vi "Populate Plugin Tree.vi"(8 "ErrorArray In":errorcluster[](array[cluster]), 10 "Userfiles Directory":path, 11 "PluginTreeRef":refnum<vi>) -> (0 "ErrorArray Out":errorcluster[](array[cluster]), 2 "All Tags":string[](array[string]), 3 "Tree Ref out":refnum<vi>)   [LabVIEW 2018]
uses:
  Controls/Plugins Tree Item Type.ctl
  <userlib>/NIST/NISTErrorLib/NISTErrorLib.lvlib
panel:
  in  "PluginTree":string(tree)
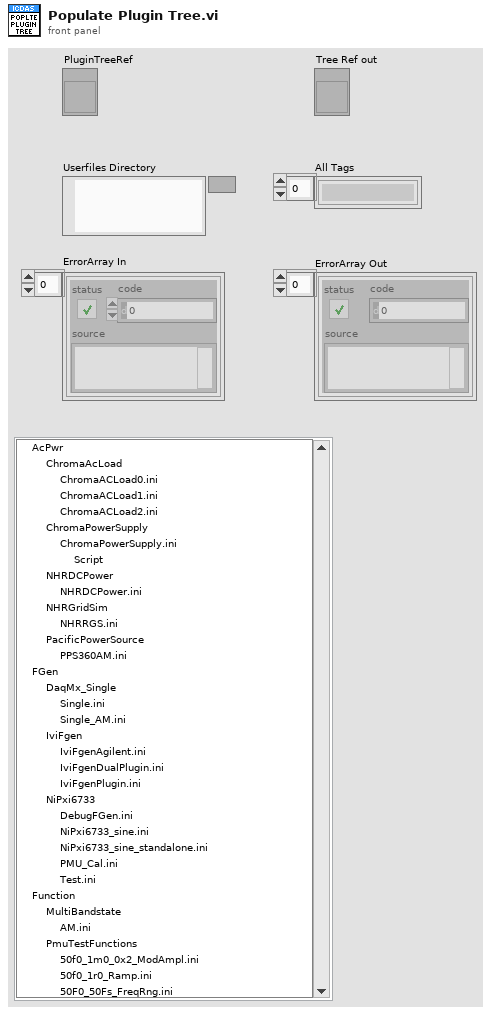
[diagram p1: front panel]
types:
  T1 = typedef "Plugins Tree Item Type.ctl" = enum16{"Plugin", "Instrument", "INI File", "INI Script"}
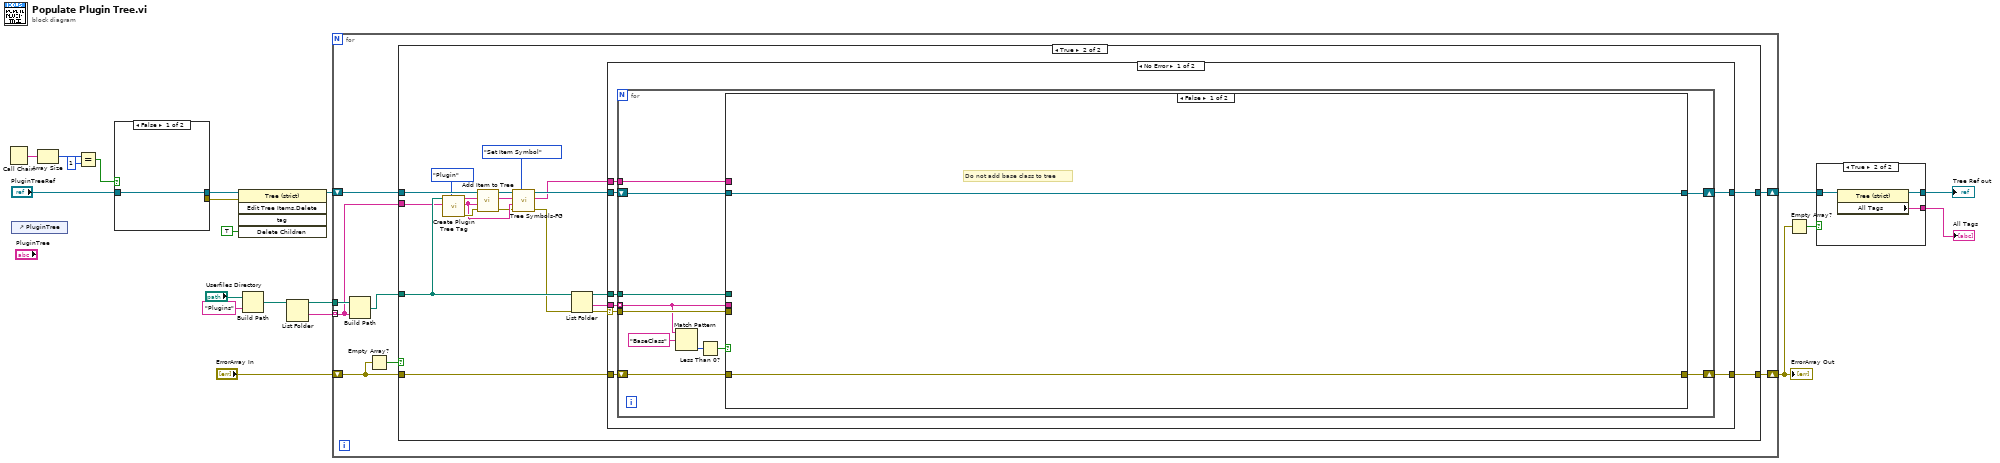
[diagram p0: block diagram]
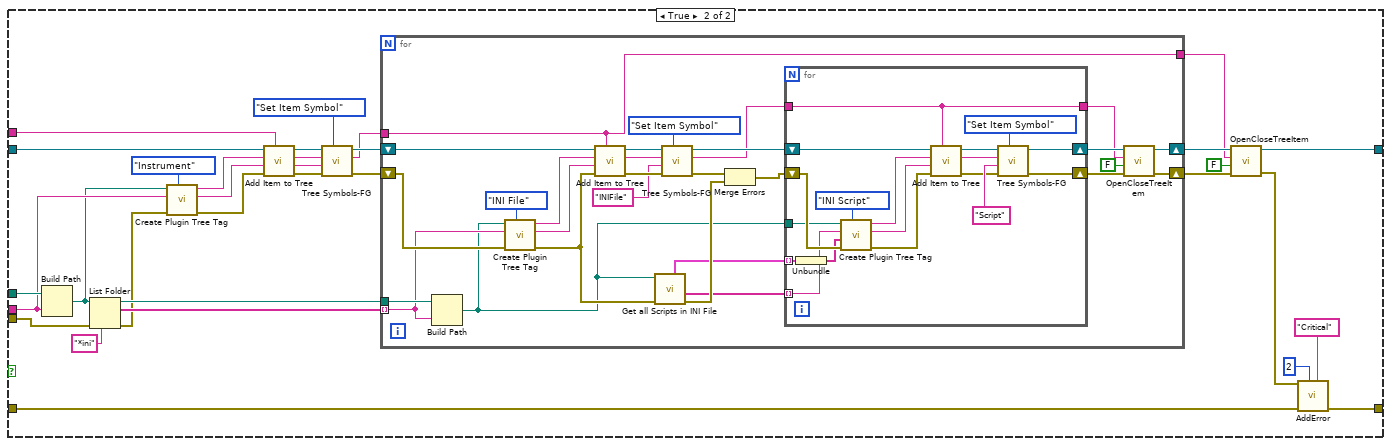
[diagram p4: hidden frame]
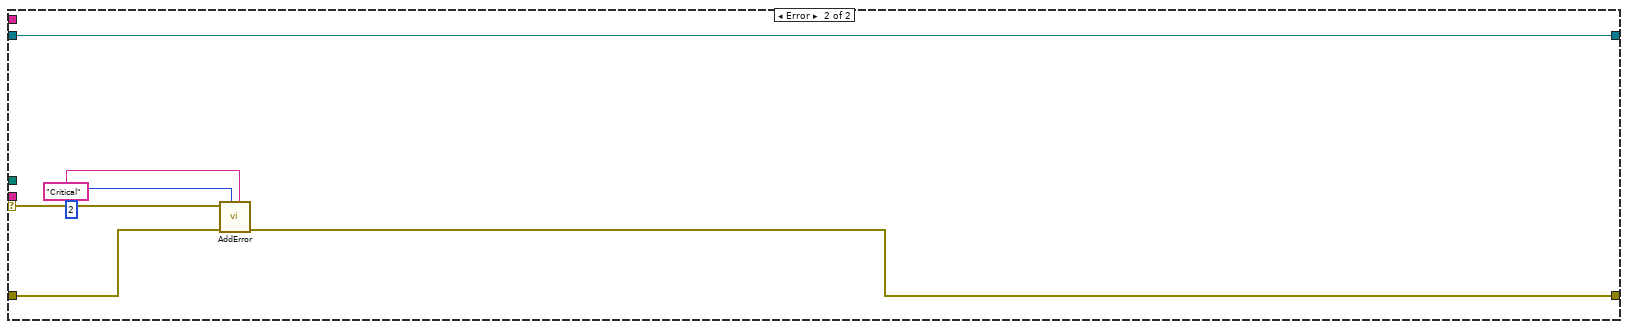
[diagram p5: hidden frame]
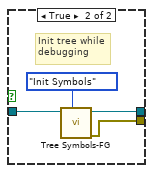
[diagram p6: hidden frame]
diagram:
  n1 = Call Chain() -> (call chain=w13:string[])
  n2 = control-ref of="PluginTree"() -> ()  [unwired: 1 out]
  n3 = Array Size(array=w13) -> (size(s)=w12:i32)
  n4 = Equal?(x=w12, y=1) -> (x = y?=w10:bool)
  n5 = case shown="False" w10 {
    tunnel: [w21 w24] -> w15
    tunnel: "PluginTreeRef" -> [w21 w23]
    tunnel: [_ w22] -> w14
    frame False {
    }
    frame True {
      # "Init tree while\ndebugging"
      n6 = call "Tree Symbols-FG.vi"("Actions"=enum16{"Init Symbols", "Set Item Symbol"}."Init Symbols", "Tree Ref"=w23) -> ("error out"=w22:errorcluster, "Tree Ref out"=w24:refnum<vi>)  [unwired: 7 in, 1 out]
    }
  }
  n7 = invoke class="Tree (strict)" method="Edit Tree Items.Delete"(reference=w15, error in=w14, "Delete Children"=TRUE ("Delete Children?")) -> (reference out=w17:refnum<vi>)  [unwired: 2 in, 4 out]
  n8 = Build Path(base path="Userfiles Directory", name or relative path="Plugins") -> (appended path=w1:path)
  n9 = List Folder(path=w1) -> (path out=w19:path, folder names=w20:string[])  [unwired: 3 in, 2 out]
  n10 = for {
    tunnel: w20 -> [w26] mode=indexing
    tunnel: w19 -> [w33]
    shift-right: [w30] -> w6
    shift-left: "ErrorArray In" -> [w31]
    shift-right: [w28] -> w8
    shift-left: w17 -> [w29]
    n11 = Build Path(base path=w33, name or relative path=w26) -> (appended path=w32:path)
    n12 = Empty Array?(array=w31) -> (empty?=w27:bool)
    n13 = case shown="True" w27 {
      tunnel: w32 -> [_ w47]
      tunnel: w31 -> [w34 w55]
      tunnel: [w34 w54] -> w30
      tunnel: w29 -> [w35 w49]
      tunnel: [w35 w50] -> w28
      tunnel: w26 -> [_ w46]
      frame False {
      }
      frame True {
        n14 = call "Create Plugin Tree Tag.vi"("ItemType"=Plugins_Tree_Item_Type."Plugin", "Name"=w46, "VISA Resource"=w47) -> ("error out"=w44:errorcluster, "Name out"=w38:string, "Tag"=w45:string)  [unwired: 6 in]
        n15 = call "Add Item to Tree.vi"("error in (no error)"=w44, "Item Name"=w38, "Item Tag"=w45, "Tree Ref"=w49) -> ("error out"=w37:errorcluster, "Item Tag out"=w40:string, "reference out"=w48:refnum<vi>)  [unwired: 4 in, 1 out]
        n16 = call "Tree Symbols-FG.vi"("Actions"=enum16{"Init Symbols", "Set Item Symbol"}."Set Item Symbol", "error in (no error)"=w37, "Symbol Name"=w38, "Item Tag"=w40, "Tree Ref"=w48) -> ("error out"=w36:errorcluster, "Item Tag out"=w39:string, "Tree Ref out"=w42:refnum<vi>)  [unwired: 4 in]
        n17 = List Folder(path=w47, error in=w36) -> (path out=w51:path, folder names=w52:string[], error out=w53:errorcluster)  [unwired: 2 in, 1 out]
        n18 = case shown="No Error" w53 {
          selector: w53 -> [w56 w159]
          tunnel: w55 -> [w61 w160]
          tunnel: [w60 w156] -> w54
          tunnel: w52 -> [w63 _]
          tunnel: w51 -> [w62 _]
          tunnel: w42 -> [w59 w155]
          tunnel: [w58 w155] -> w50
          tunnel: w39 -> [w57 _]
          frame No Error {
            n19 = for {
              tunnel: w63 -> [w67] mode=indexing
              tunnel: w62 -> [w74]
              shift-right: [w72] -> w60
              shift-left: w61 -> [w73]
              shift-right: [w68] -> w58
              shift-left: w59 -> [w71]
              tunnel: w57 -> [w70]
              tunnel: w56 -> [w69]
              n20 = Match Pattern(string=w67, regular expression="BaseClass") -> (offset past match=w65:i32)  [unwired: 1 in, 3 out]
              n21 = Less Than 0?(x=w65) -> (x < 0?=w64:bool)
              n22 = case shown="False" w64 {
                tunnel: w74 -> [_ w106]
                tunnel: w73 -> [w76 w104]
                tunnel: [w76 w103] -> w72
                tunnel: w71 -> [w75 w100]
                tunnel: w70 -> [_ w99]
                tunnel: w67 -> [_ w98]
                tunnel: w69 -> [_ w91]
                tunnel: [w75 w81] -> w68
                frame False {
                  # "Do not add base class to tree"
                }
                frame True {
                  n23 = Build Path(base path=w106, name or relative path=w98) -> (appended path=w97:path)
                  n24 = List Folder(path=w97, pattern="*ini", error in=w91) -> (path out=w105:path, filenames=w107:string[], error out=w90:errorcluster)  [unwired: 1 in, 1 out]
                  n25 = call "Create Plugin Tree Tag.vi"("ItemType"=Plugins_Tree_Item_Type."Instrument", "error in (no error)"=w90, "Name"=w98, "VISA Resource"=w97) -> ("error out"=w93:errorcluster, "Name out"=w94:string, "Tag"=w95:string)  [unwired: 5 in]
                  n26 = call "Add Item to Tree.vi"("Parent Tag"=w99, "error in (no error)"=w93, "Item Name"=w94, "Item Tag"=w95, "Tree Ref"=w100) -> ("error out"=w92:errorcluster, "Item Name out"=w83:string, "Item Tag out"=w86:string, "reference out"=w88:refnum<vi>)  [unwired: 3 in]
                  n27 = call "Tree Symbols-FG.vi"("Actions"=enum16{"Init Symbols", "Set Item Symbol"}."Set Item Symbol", "error in (no error)"=w92, "Symbol Name"=w83, "Item Tag"=w86, "Tree Ref"=w88) -> ("error out"=w89:errorcluster, "Item Tag out"=w85:string, "Tree Ref out"=w87:refnum<vi>)  [unwired: 4 in]
                  n28 = for {
                    tunnel: w107 -> [w132] mode=indexing
                    tunnel: w105 -> [w133]
                    tunnel: w85 -> [w109]
                    shift-right: [w112] -> w82
                    shift-left: w87 -> [w130]
                    shift-right: [w114] -> w79
                    shift-left: w89 -> [w134]
                    tunnel: [w109] -> w80
                    n29 = Build Path(base path=w133, name or relative path=w132) -> (appended path=w118:path)
                    n30 = call "Create Plugin Tree Tag.vi"("ItemType"=Plugins_Tree_Item_Type."INI File", "error in (no error)"=w134, "Name"=w132, "VISA Resource"=w118) -> ("error out"=w123:errorcluster, "Name out"=w136:string, "Tag"=w131:string)  [unwired: 5 in]
                    n31 = call "Add Item to Tree.vi"("Parent Tag"=w109, "error in (no error)"=w123, "Item Name"=w136, "Item Tag"=w131, "Tree Ref"=w130) -> ("error out"=w129:errorcluster, "Item Tag out"=w127:string, "reference out"=w128:refnum<vi>)  [unwired: 3 in, 1 out]
                    n32 = call "Get all Scripts in INI File.vi"("error in (no error)"=w123, "configuration file path"=w118) -> ("error out"=w121:errorcluster, "All Scipts w/o *"=w116:string[], "Scripts"=w115:cluster{string[]}[])  [unwired: 6 in, 1 out]
                    n33 = call "Tree Symbols-FG.vi"("Actions"=enum16{"Init Symbols", "Set Item Symbol"}."Set Item Symbol", "error in (no error)"=w129, "Symbol Name"="INIFile", "Item Tag"=w127, "Tree Ref"=w128) -> ("error out"=w122:errorcluster, "Item Tag out"=w117:string, "Tree Ref out"=w124:refnum<vi>)  [unwired: 4 in]
                    n34 = Merge Errors(w122, w121) -> (w119:errorcluster)
                    n35 = for {
                      shift-right: [w144] -> w113
                      shift-left: w124 -> [w147]
                      shift-right: [w146] -> w120
                      shift-left: w119 -> [w145]
                      tunnel: w118 -> [w143]
                      tunnel: w117 -> [w140]
                      tunnel: w116 -> [w137] mode=indexing
                      tunnel: w115 -> [w142] mode=indexing
                      tunnel: [w140] -> w111
                      n36 = Unbundle(w142) -> (w141:string[])
                      n37 = call "Create Plugin Tree Tag.vi"("ItemType"=Plugins_Tree_Item_Type."INI Script", "error in (no error)"=w145, "Script"=w141, "Name"=w137, "VISA Resource"=w143) -> ("error out"=w154:errorcluster, "Name out"=w138:string, "Tag"=w149:string)  [unwired: 4 in]
                      n38 = call "Add Item to Tree.vi"("Parent Tag"=w140, "error in (no error)"=w154, "Item Name"=w138, "Item Tag"=w149, "Tree Ref"=w147) -> ("error out"=w150:errorcluster, "Item Tag out"=w139:string, "reference out"=w151:refnum<vi>)  [unwired: 3 in, 1 out]
                      n39 = call "Tree Symbols-FG.vi"("Actions"=enum16{"Init Symbols", "Set Item Symbol"}."Set Item Symbol", "error in (no error)"=w150, "Symbol Name"="Script", "Item Tag"=w139, "Tree Ref"=w151) -> ("error out"=w146:errorcluster, "Tree Ref out"=w144:refnum<vi>)  [unwired: 4 in, 1 out]
                    }
                    n40 = call "OpenCloseTreeItem.vi"("error in (no error)"=w120, "Open?"=FALSE, "Item Tag in"=w111, "TreeControl in"=w113) -> ("error out"=w114:errorcluster, "TreeControl out"=w112:refnum<vi>)  [unwired: 5 in, 1 out]
                  }
                  n41 = call "OpenCloseTreeItem.vi"("error in (no error)"=w79, "Open?"=FALSE, "Item Tag in"=w80, "TreeControl in"=w82) -> ("error out"=w77:errorcluster, "TreeControl out"=w81:refnum<vi>)  [unwired: 5 in, 1 out]
                  n42 = call <userlib>:"AddError.vi"("Severity"="Critical", "Priority"=u8 2, "ErrorArray In"=w104, "error in (no error)"=w77) -> ("ErrorArray Out"=w103:errorcluster[])  [unwired: 6 in, 1 out]
                }
              }
            }
          }
          frame Error {
            n43 = call <userlib>:"AddError.vi"("Severity"="Critical", "Priority"=u8 2, "ErrorArray In"=w160, "error in (no error)"=w159) -> ("ErrorArray Out"=w156:errorcluster[])  [unwired: 6 in, 1 out]
          }
        }
      }
    }
  }
  "ErrorArray Out" <- w6
  n44 = Empty Array?(array=w6) -> (empty?=w7:bool)
  n45 = case shown="True" w7 {
    tunnel: w8 -> [w161 w164]
    tunnel: [w161 w163] -> w5
    tunnel: [_ w162] -> w4
    frame False {
    }
    frame True {
      n46 = property class="Tree (strict)"(reference=w164) -> (reference out=w163:refnum<vi>, "All Tags"=w162:string[])  [unwired: 1 in, 1 out]
    }
  }
  "Tree Ref out" <- w5
  "All Tags" <- w4
